vi "StepperMotorXYControl.vi"() -> ()   [LabVIEW 2011]
uses:
  Main/GlobalVariables.vi
panel:
  in  "Y Channel value":dbl
  in  "X Channel value":dbl
  in  "System no.":i32=4
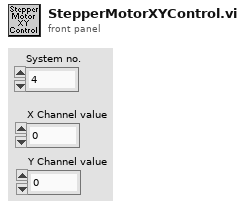
[diagram p1: front panel]
types:
  T1 = enum16{"Interface", "Digital TTL Control - level controlled", "Digital TTL Control - edge controlled", "Digital TTL Control - quadrature controlled", "Analog input - linear", "Analog input - level controlled"}[]
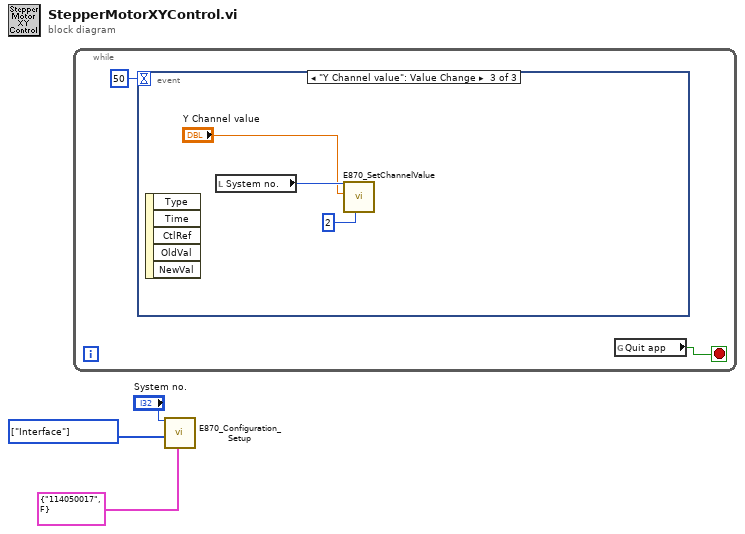
[diagram p0: block diagram]
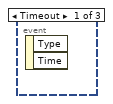
[diagram p2: hidden frame]
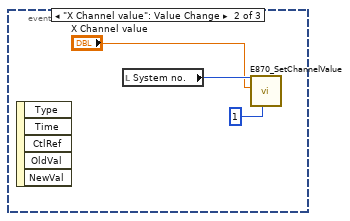
[diagram p3: hidden frame]
diagram:
  w2 = T1 [enum."Interface"] items=["Interface", "Digital TTL Control - level controlled", "Digital TTL Control - edge controlled", "Digital TTL Control - quadrature controlled", "Analog input - linear", "Analog input - level controlled"] ("Select\nCommand mode")
  n1 = while {
    stop <- w5 stop-if-true
    n2 = event shown="[2] \"Y Channel value\": Value Change" {
      selector: _ -> [_ _ _]
      dyn-events: _ -> [_ _ _]
      timeout: 50 -> [_ _ _]
      event Timeout {
        n3 = event-data() -> ()  [unwired: 1 in, 2 out]
      }
      event "X Channel value": Value Change {
        n4 = event-data() -> ()  [unwired: 1 in, 5 out]
        n5 = local read "System no."() -> (w8:i32)
        n6 = call "E870_SetChannelValue.vi"("Channel #"=1, "# Steps"="X Channel value", "System no."=w8) -> ()  [unwired: 9 in]
      }
      event "Y Channel value": Value Change {
        n7 = event-data() -> ()  [unwired: 1 in, 5 out]
        n8 = local read "System no."() -> (w11:i32)
        n9 = call "E870_SetChannelValue.vi"("Channel #"=2, "# Steps"="Y Channel value", "System no."=w11) -> ()  [unwired: 9 in]
      }
    }
    n10 = global read "GlobalVariables.vi" "Quit app"() -> (w5:bool)
  }
  n11 = call "E870_Configuration_Setup.vi"("System no."="System no.", "Select\nCommand mode"=w2, "USB settings"=cluster{"S/N":string, "USB Search?":bool} {"S/N"="114050017", "USB Search?"=FALSE}) -> ()  [unwired: 10 in, 7 out]
